vi "Decorate.vi"(10 "Actor":refnum<class "Actor.lvclass">, 11 "TEMPLATE jettl in":refnum<class "TEMPLATE jettl.lvclass">) -> (3 "TEMPLATE jettl out":refnum<class "TEMPLATE jettl.lvclass">)   [LabVIEW 2021, in "_Template.lvlib" / "Templates.lvlib" / "TEMPLATE jettl.lvlib" / "TEMPLATE jettl.lvclass"]
uses:
  TEMPLATE jettl.lvclass
  TEMPLATE jettl.lvclass/TEMPLATE jettl.ctl
  jettl/jettl/Actor/Actor/Actor.lvclass
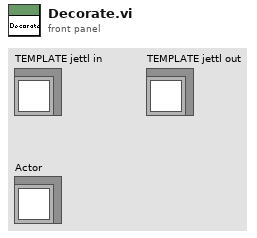
[diagram p1: front panel]
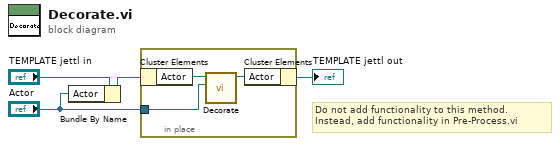
[diagram p0: block diagram]
diagram:
  # "Do not add functionality to this method. Instead, add functionality in Pre-Process.vi"
  n1 = Bundle By Name(cluster="TEMPLATE jettl in", "Actor"="Actor") -> (w3:refnum<class "TEMPLATE jettl.lvclass">)
  n2 = in-place {
    in-place-border: "Actor" -> [w5]
    n3 = in-place-cluster #1(w3) -> ("Actor"=w7:refnum<class "Actor.lvclass">)
    n4 = call-dynamic "Decorate.vi"("Actor"=w5, "Actor in"=w7) -> ("Actor out"=w6:refnum<class "Actor.lvclass">)  [unwired: 9 in]
    n5 = in-place-cluster #1("Actor"=w6) -> (→"TEMPLATE jettl out":refnum<class "TEMPLATE jettl.lvclass">)
  }
